vi "Query Power Measurement Parameter Predefined Sets Catalog.vi"(8 "error in (no error)":errorcluster, 10 "Instance (1)":i32=1, 11 "VISA resource name":refnum<visa-resource-name>) -> (0 "error out":errorcluster, 2 "Catalog":string, 3 "VISA resource name out":refnum<visa-resource-name>)   [LabVIEW 2020, in "Rohde&Schwarz CMXP GPRF.lvlib"]
doc: "Gets a comma/separated list of predefined parameter sets that can be loaded as parameter set in retriggered list mode.\n\nAttribute:\nRSCMXPGPRF_ATTR_POWER_MEASUREMENT_PARAMETER_SETS_CATALOG\n\nRemote-control command:\nCONFigure:GPRF:MEAS<i>:POWer:PSET:CATalog:PDEFset?"
uses:
  <instrlib>/Rohde&Schwarz CMXP GPRF/Rohde&Schwarz CMXP GPRF.lvlib
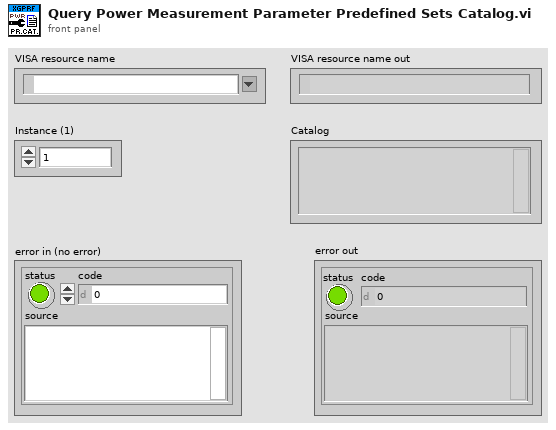
[diagram p1: front panel]
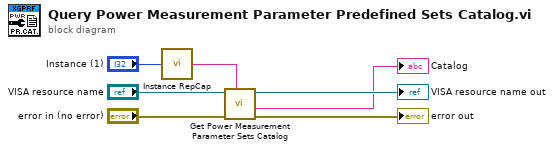
[diagram p0: block diagram]
diagram:
  n1 = call <instrlib>:"Instance RepCap.vi"("Instance in"="Instance (1)") -> ("Instance out"=w7:string)
  n2 = call "Get Power Measurement Parameter Sets Catalog"("Repeated Capabilities"=w7, "error in (no error)"="error in (no error)", "instrument handle"="VISA resource name") -> ("error out"=→"error out":errorcluster, "Power Measurement Parameter Sets Catalog"=→"Catalog":string, "instrument handle out"=→"VISA resource name out":refnum<visa-resource-name>)  [unwired: 6 in]
